vi "dfd_DFXP_DFXP to Double (scaler).vi"(11 "Value in":T1={"value"=0, "wl"=0, "iwl"=0, "Signed"=TRUE} {"value" format="%.0x"}) -> (3 "DBL":dbl)   [LabVIEW 2017, in "NI_DigFilter_FXP.lvlib"]
uses:
  <vilib>/addons/Digital Filter Design/NI_DigFilter_FXP.lvlib
  <vilib>/addons/Digital Filter Design/_Objects.llb/dfd_DFXP Data Type (scaler).ctl
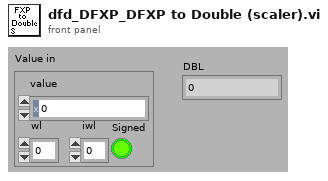
[diagram p1: front panel]
types:
  T1 = typedef "dfd_DFXP Data Type (scaler).ctl" = cluster{"value":i64, "wl":i16, "iwl":i16, "Signed":bool}
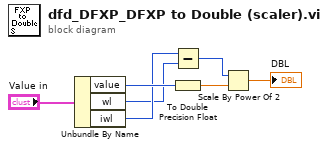
[diagram p0: block diagram]
diagram:
  n1 = Unbundle By Name("Value in") -> ("value"=w4:i64, "wl"=w1:i16, "iwl"=w2:i16)
  n2 = Subtract(x=w2, y=w1) -> (x-y=w3:i16)
  n3 = To Double Precision Float(number=w4) -> (double precision float=w5:dbl)
  n4 = Scale By Power Of 2(n=w3, x=w5) -> (x*2^n=→"DBL":dbl)
